vi "humbleBundle.vi"() -> ()   [LabVIEW 2016]
panel:
  out "Slide":u8(slide) scale=0.0..100.0
  out "Numeric 2":dbl
  out "Numeric":dbl
  in  "stop":bool
  in  "Numeric 4":dbl
  in  "Numeric 3":dbl
  in  "Color #":u32(colorbox)
  in  "string name":string
  in  "other Boolean":bool
  in  "oj Button":bool
  in  "Boolean 1":bool
  # "This is a comment!"
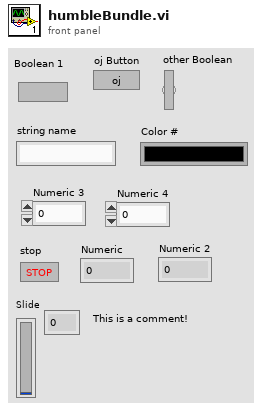
[diagram p1: front panel]
types:
  T1 = cluster{"Boolean":bool, "Boolean 1":bool, "other Boolean":bool, "string name":string, "Color #s":u32, "Numeric 3":dbl, "Numeric 4":dbl}
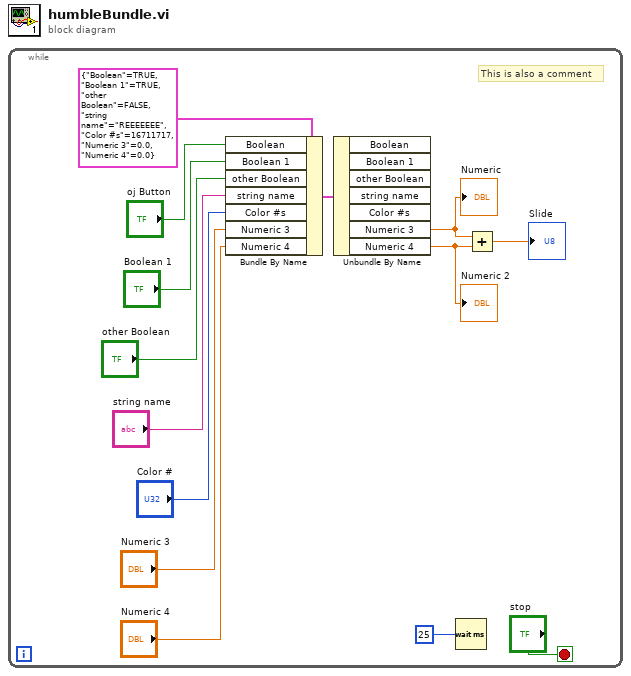
[diagram p0: block diagram]
diagram:
  # "This is also a comment"
  n1 = while {
    stop <- "stop" stop-if-true
    n2 = Bundle By Name(cluster=T1 {"Boolean"=TRUE, "Boolean 1"=TRUE, "other Boolean"=FALSE, "string name"="REEEEEEE", "Color #s"=16711717, "Numeric 3"=0.0, "Numeric 4"=0.0}, "Boolean"="oj Button", "Boolean 1"="Boolean 1", "other Boolean"="other Boolean", "string name"="string name", "Color #s"="Color #", "Numeric 3"="Numeric 3", "Numeric 4"="Numeric 4") -> (w5:T1)
    n3 = Unbundle By Name(w5) -> ("Numeric 3"=w3:dbl, "Numeric 4"=w2:dbl)  [unwired: 5 out]
    "Numeric" <- w3
    "Numeric 2" <- w2
    n4 = Wait (ms)(milliseconds to wait=25) -> ()  [unwired: 1 out]
    n5 = Add(x=w3, y=w2) -> (x+y=→"Slide":dbl)
  }
